vi "Display Message Loop.vi"(7 "Message Queues":T1, 8 "error in (no error)":errorcluster, 9 "XYGraph Refnum":refnum<vi>, 10 "Calibration Refnum":refnum<vi>, 11 "Design Results Refnum":refnum<vi>) -> (0 "error out":errorcluster)   [LabVIEW 2025]
uses:
  support/Message Queue/All Message Queues.ctl
  support/Message Queue/Message Cluster.ctl
  controls/Design_Results.ctl
  controls/Calibration_Data.ctl
  controls/Constants.ctl
  controls/Designing Loop Enum.ctl
  support/Message Queue/Message Queue.lvlib
panel:
  # "Simulator Fit"
  # "Empirical Fit"
  # "="
  # "P"
  # "* X"
  # "P"
  # "="
  # "* X"
  # "drop"
  # "drop"
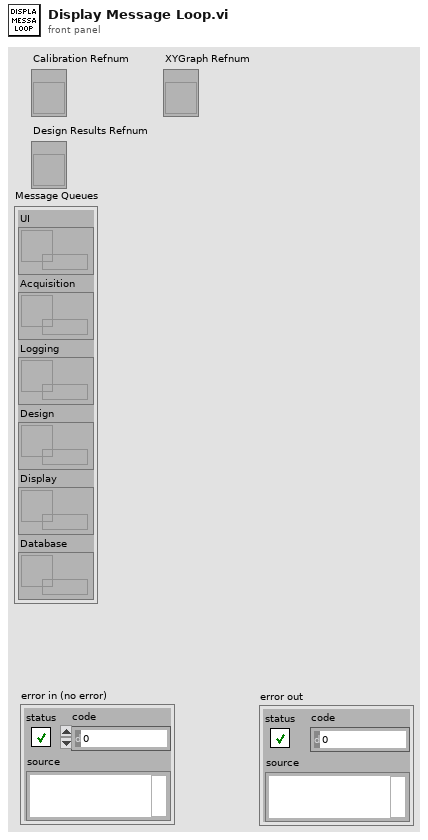
[diagram p1: front panel]
types:
  T1 = typedef "Message Queue.lvlib/All Message Queues.ctl" = cluster{"UI":refnum<queue>, "Acquisition":refnum<queue>, "Logging":refnum<queue>, "Design":refnum<queue>, "Display":refnum<queue>, "Database":refnum<queue>}
  T2 = typedef "Calibration_Data.ctl" = cluster{"Flow Rate (LBM/MIN)":dbl, "Pressure Ambient (PSIA)":dbl, "Pressure Inlet (PSIG)":dbl, "Pressure Tap (PSIG)":dbl, "Temperature Ambient (DEG F)":dbl, "Temperature Inlet (DEG F)":dbl, "Temperature Tap (DEG F)":dbl}
  T3 = typedef "Design_Results.ctl" = cluster{"Design Results":cluster{"Model Validation: Simulated vs. Empirical Airflow Data":cluster{dbl[], dbl[]}[], "Amplitude - Empirical":string, "Power - Empirical":string, "Amplitude - Sim":string, "Power - Sim":string, "Flow Type":u32, "Optimized Inlet \nOrifice Diameter (in)":dbl, "Flow Type Name":string}}
  T4 = typedef "Designing Loop Enum.ctl" = enum16{"Output New Results", "Start"}
  T5 = typedef "Constants.ctl" = cluster{"P_amb (psia)":dbl, "T_in (Deg F)":dbl, "R_air (ft*lbf)/(lbm*R)":dbl, "g_c (lbm*ft)/(lbf*s^2)":dbl, "specific heat ratio":dbl, "Viscousity (lbm)/(ft*s)":dbl, "Cd":dbl, "Mass Flow (lbm/min) vs. Pressure Drop (inH2O) - Real Data":dbl[][]}
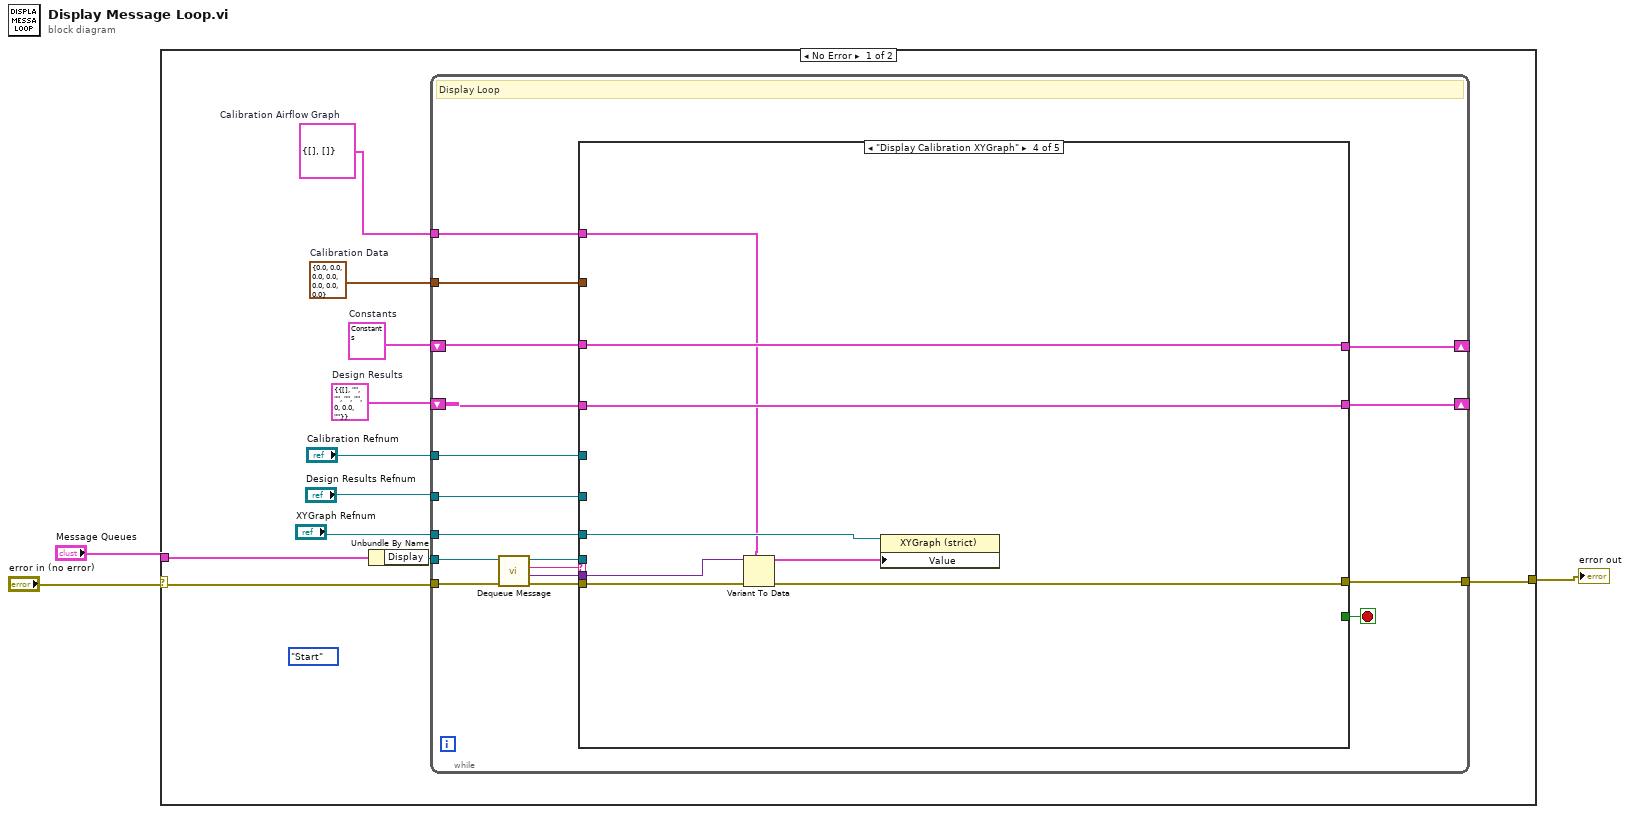
[diagram p0: block diagram]
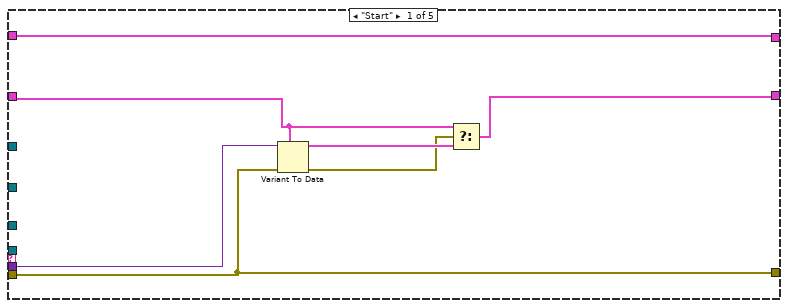
[diagram p2: hidden frame]
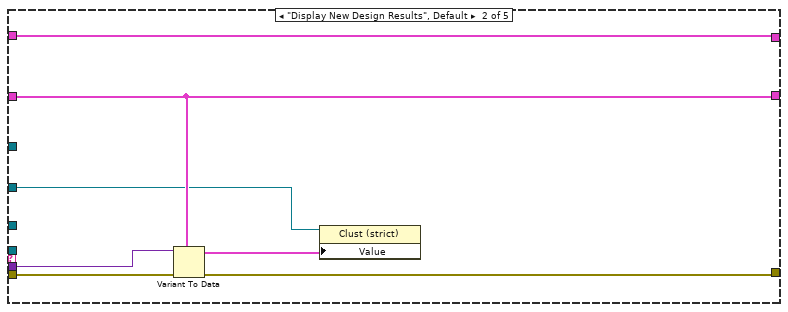
[diagram p3: hidden frame]
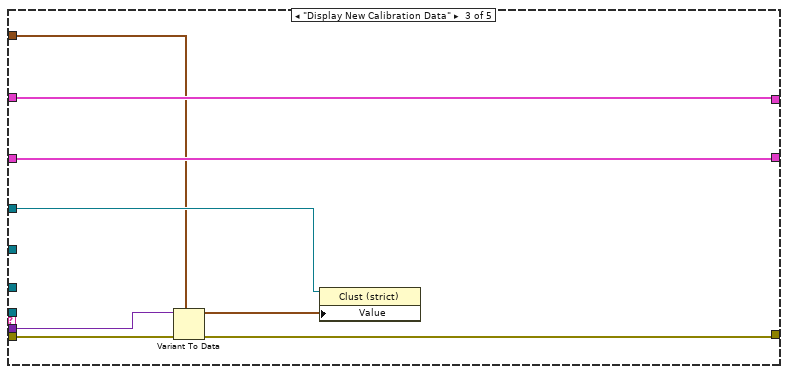
[diagram p4: hidden frame]
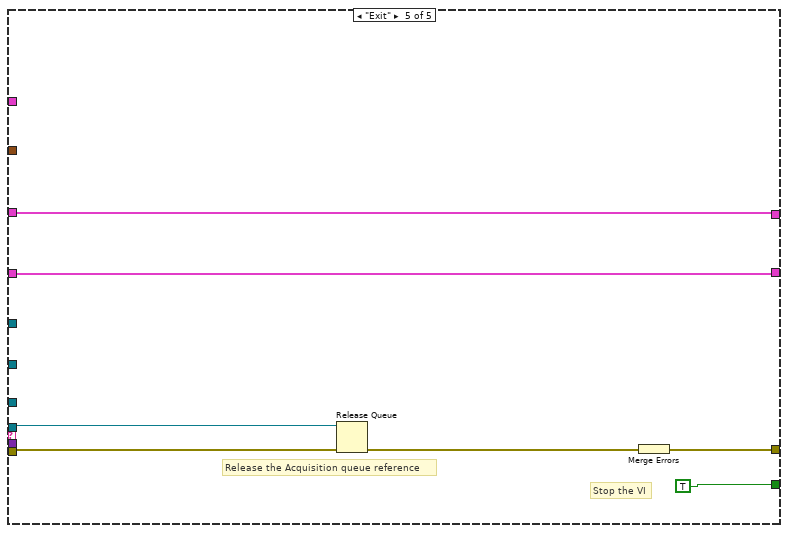
[diagram p5: hidden frame]
diagram:
  n1 = case shown="No Error" "error in (no error)" {
    selector: "error in (no error)" -> [w12 w69]
    tunnel: "Message Queues" -> [w14 _]
    tunnel: [w11 w69] -> w1
    frame No Error {
      w5 = cluster{dbl[], dbl[]} {[], []}  # Calibration Airflow Graph
      w6 = T2 {"Flow Rate (LBM/MIN)"=0.0, "Pressure Ambient (PSIA)"=0.0, "Pressure Inlet (PSIG)"=0.0, "Pressure Tap (PSIG)"=0.0, "Temperature Ambient (DEG F)"=0.0, "Temperature Inlet (DEG F)"=0.0, "Temperature Tap (DEG F)"=0.0}  # Calibration Data
      w9 = T3 {"Design Results"={"Model Validation: Simulated vs. Empirical Airflow Data"=[], "Amplitude - Empirical"="", "Power - Empirical"="", "Amplitude - Sim"="", "Power - Sim"="", "Flow Type"=0, "Optimized Inlet \nOrifice Diameter (in)"=0.0, "Flow Type Name"=""}}  # Design Results
      (unwired) Designing_Loop_Enum."Start"
      w10 = T5 {"P_amb (psia)"=14.7, "T_in (Deg F)"=70.0, "R_air (ft*lbf)/(lbm*R)"=53.35, "g_c (lbm*ft)/(lbf*s^2)"=32.17, "specific heat ratio"=1.4, "Viscousity (lbm)/(ft*s)"=1.21e-05, "Cd"=0.61, "Mass Flow (lbm/min) vs. Pressure Drop (inH2O) - Real Data"=[[0.5, 0.015], [1.0, 0.062], [1.5, 0.141], [2.0, 0.252], [2.5, 0.395], [3.5, 0.778]]}  # Constants
      n2 = Unbundle By Name(w14) -> ("Display"=w13:refnum<queue>)
      n3 = while {
        tunnel: w13 -> [w25]
        tunnel: w12 -> [w31]
        tunnel: [w30] -> w11
        shift-right: [w28] -> _
        shift-left: w9 -> [w29]
        shift-right: [w26] -> _
        shift-left: w10 -> [w27]
        tunnel: "Design Results Refnum" -> [w19]
        tunnel: "Calibration Refnum" -> [w18]
        tunnel: w6 -> [w17]
        tunnel: "XYGraph Refnum" -> [w16]
        tunnel: w5 -> [w15]
        stop <- w20 stop-if-true
        # "Display Loop"
        n4 = call "Dequeue Message.vi"("error in (no error)"=w31, "Message Queue"=w25) -> ("error out"=w24:errorcluster, "Message Data"=w22:variant, "Message"=w23:string, "dup Message Queue"=w21:refnum<queue>)  [unwired: 6 in]
        n5 = case shown="\"Display Calibration XYGraph\"" w23 {
          tunnel: [w35 w42 w50 w58 w66] -> w30
          tunnel: w29 -> [w38 w41 w49 w57 w63]
          tunnel: [w37 w41 w49 w57 w63] -> w28
          tunnel: w27 -> [w36 w45 w53 w61 w62]
          tunnel: [w36 w45 w53 w61 w62] -> w26
          tunnel: w24 -> [w35 w43 w51 w59 w65]
          tunnel: w22 -> [w32 w44 w52 w60 _]
          tunnel: w21 -> [_ _ _ _ w64]
          tunnel: [_ _ _ _ TRUE] -> w20
          tunnel: w19 -> [_ w40 _ _ _]
          tunnel: w18 -> [_ _ w48 _ _]
          tunnel: w17 -> [_ _ w47 _ _]
          tunnel: w16 -> [_ _ _ w56 _]
          tunnel: w15 -> [_ _ _ w55 _]
          frame "Start" {
            n6 = Variant To Data(error in=w35, type=w38, Variant=w32) -> (data=w34:T3, error out=w33:errorcluster)
            n7 = Select(t=w38, s=w33, f=w34) -> (s? t:f=w37:T3)
          }
          frame "Display New Design Results", Default {
            n8 = Variant To Data(error in=w43, type=w41, Variant=w44) -> (data=w39:T3, error out=w42:errorcluster)
            n9 = property class="Clust (strict)"(reference=w40, "Value"=w39) -> ()  [unwired: 1 in, 2 out]
          }
          frame "Display New Calibration Data" {
            n10 = Variant To Data(error in=w51, type=w47, Variant=w52) -> (data=w46:T2, error out=w50:errorcluster)
            n11 = property class="Clust (strict)"(reference=w48, "Value"=w46) -> ()  [unwired: 1 in, 2 out]
          }
          frame "Display Calibration XYGraph" {
            n12 = Variant To Data(error in=w59, type=w55, Variant=w60) -> (data=w54:cluster{dbl[], dbl[]}, error out=w58:errorcluster)
            n13 = property class="XYGraph (strict)"(reference=w56, "Value"=w54) -> ()  [unwired: 1 in, 2 out]
          }
          frame "Exit" {
            # "Release the Acquisition queue reference"
            # "Stop the VI"
            n14 = Release Queue(queue=w64, error in (no error)=w65) -> (error out=w68:errorcluster)  [unwired: 1 in, 2 out]
            n15 = Merge Errors(w68) -> (w66:errorcluster)
          }
        }
      }
    }
    frame Error {
    }
  }
  "error out" <- w1
